vi "总氮质控流程.vi"(6 "队列输入TN":refnum<queue>, 9 "总氮":bool, 10 "总氮量程切换":enum32{"H", "L", "AUTO"}(ring)=enum."AUTO") -> (2 "总氮中断报警":bool, 3 "布尔":bool)   [LabVIEW 2016]
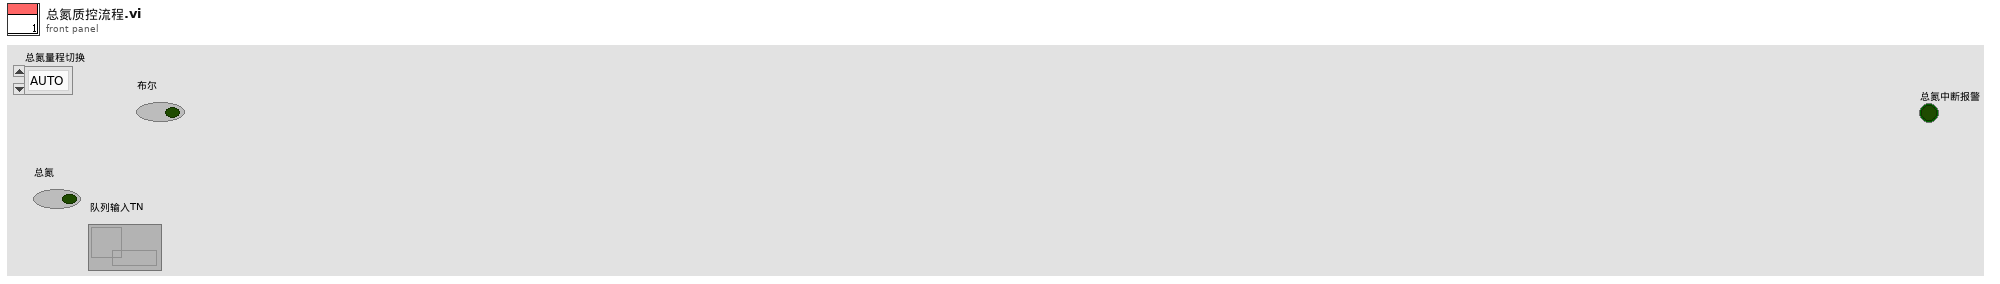
[diagram p1: front panel]
types:
  T1 = enum16{"待机", "启动氨氮水样", "氨氮测量中", "启动氨氮加标", "启动氨氮加标回收", "氨氮加标回收测量中", "启动总氮水样", "总氮测量中", "启动总氮加标", "启动总氮加标回收", "总氮加标回收测量中", "启动总磷水样", "总磷水样测量中", "启动总磷加标", "启动总磷加标回收", "总磷加标回收测量中", "结束"}
  T2 = cluster{"站号":u16, "量程切换":enum32{"H", "L", "AUTO"}, "控制命令":enum16{"启动测量", "标样核查", "零点核查", "跨度核查", "空白测试", "平行样测试", "加标回收", "空白校准", "标样校准", "初始化（清洗）", "停止测试", "仪器重启", "校时", "模式设置", "测量间隔设置"}, "模式设置":enum16{"待机", "连续模式", "周期模式", "定点模式", "受控模式", "手动模式"}, "测量间隔":u16}
  T3 = cluster{"时间标识":timestamp, "设备":string, "日志信息":string}
  T4 = cluster{"系统时间":timestamp, "工作状态":enum16{"空闲", "水样测试", "标样核查", "零点核查", "跨度核查", "空白测试", "平行样测试", "加标回收", "空白校准", "标样校准", "初始化（清洗）"}, "测量模式":enum16{"待机", "连续模式", "周期模式", "定点模式", "受控模式", "手动模式"}, "告警代码":enum16{"无告警", "缺试剂告警", "缺水样告警", "缺蒸馏水告警", "缺标液告警", "仪表漏液告警", "标定异常告警", "超量程告警", "加热异常", "低试剂预警", "超上限告警", "超下限告警", "仪表内部其他异常", "滴定异常告警", "电极异常告警", "量程切换告警", "参数设置告警", "PH电极电位异常", "电导率电极异常", "浊度光度异常", "溶解氧电极异常", "溶解氧光强异常", "温度异常告警", "PH异常告警", "溶解氧异常告警", "电导率异常告警", "浊度异常告警", "叶绿素异常告警", "藻密度异常告警", "蓝绿藻异常告警", "ORP异常告警", "氨氮异常告警", "清洁刷异常告警", "SD卡异常告警", "蓝牙异常告警", "Wifi异常告警", "流程异常告警"}, "故障代码":enum16{"无故障", "电机故障", "温度故障", "通讯故障", "滴定故障"}, "日志代码":u16, "软件版本":u16, "F0":sgl, "F1":sgl, "F2":sgl, "F3":sgl, "T":sgl, "H":sgl, "id":u16, "flowid":u16, "量程":u16, "总磷控温温度1":sgl, "营养盐控温温度2":sgl, "ADC":sgl}
  T5 = enum16{"空闲", "水样测试", "标样核查", "零点核查", "跨度核查", "空白测试", "平行样测试", "加标回收", "空白校准", "标样校准", "初始化（清洗）"}
  T6 = cluster{"因子编码":u32, "单位":u16, "标样参考值":sgl, "水样数据时间":timestamp, "水样实测值":sgl, "水样数据标识":string, "标样数据时间":timestamp, "标样实测值":sgl, "标样数据标识":string, "空白数据时间":timestamp, "空白实测值":sgl, "空白数据标识":string, "零点核查数据时间":timestamp, "零点核查实测值":sgl, "零点核查数据标识":string, "跨度核查数据时间":timestamp, "跨度核查实测值":sgl, "跨度核查数据标识":string, "加标回收数据时间":timestamp, "加标回收实测值":sgl, "加标回收数据标识":string, "平行样数据时间":timestamp, "平行样实测值":sgl, "平行样数据标识":string}
  T7 = cluster{"量程":dbl, "检出限":dbl, "加标前水样浓度":dbl, "加标后水样浓度":dbl, "加标水杯定容体积":dbl, "加标母液浓度":dbl, "加标体积":dbl, "加标回收率":dbl}
  T8 = cluster{"氨氮":u8, "总磷":u8, "总氮":u8, "CODMn":u8, "CODCr":u8}
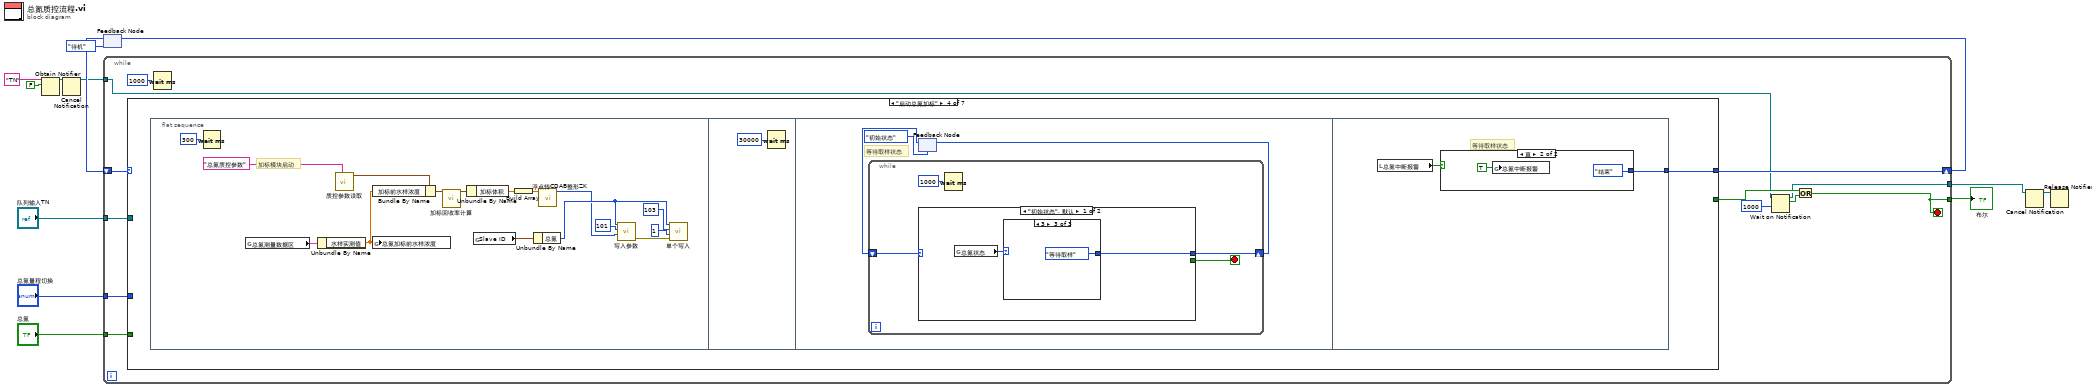
[diagram p0: block diagram]
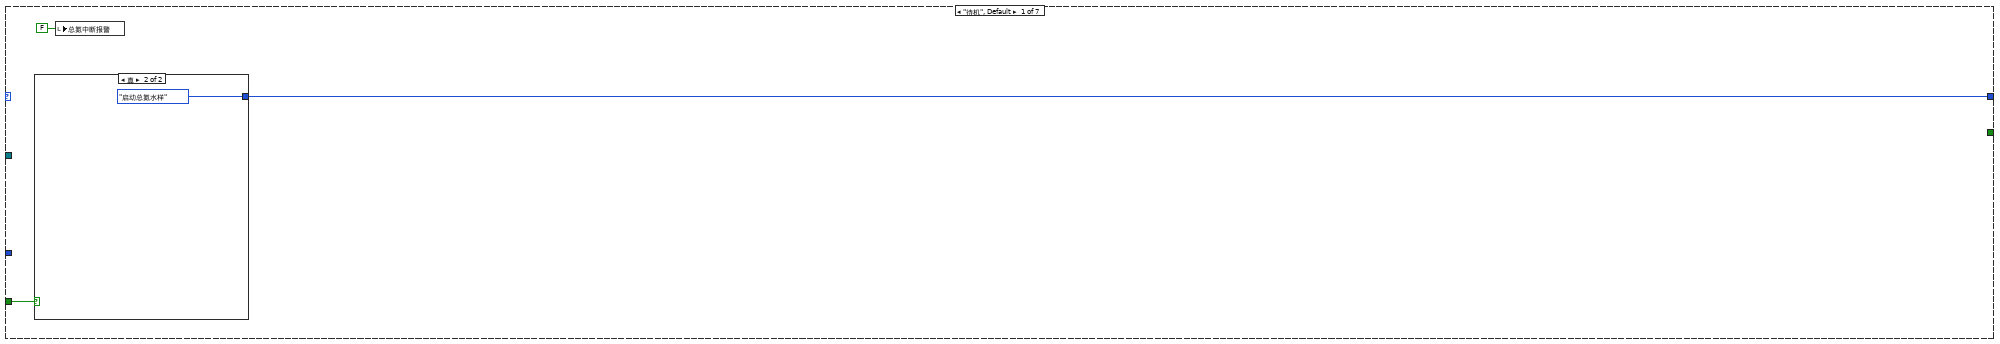
[diagram p2: hidden frame]
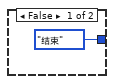
[diagram p3: hidden frame]
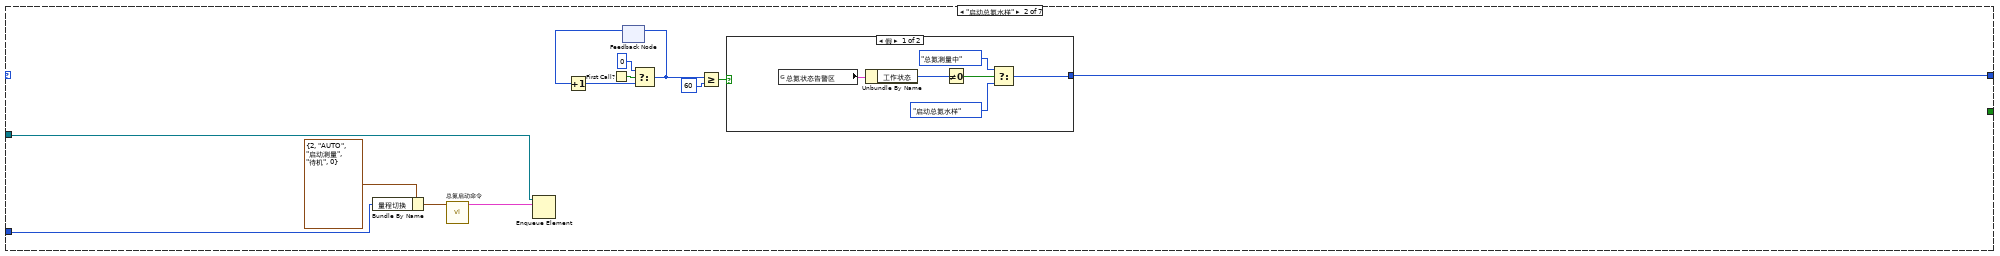
[diagram p4: hidden frame]
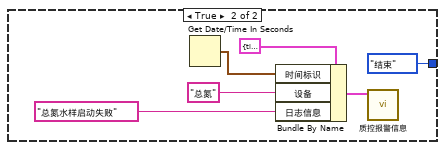
[diagram p5: hidden frame]
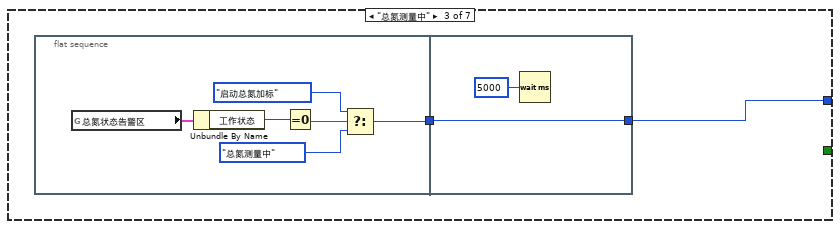
[diagram p6: hidden frame]
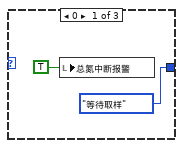
[diagram p7: hidden frame]
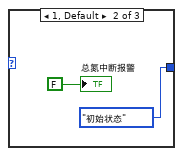
[diagram p8: hidden frame]
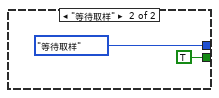
[diagram p9: hidden frame]
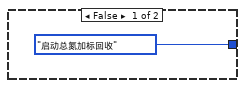
[diagram p10: hidden frame]
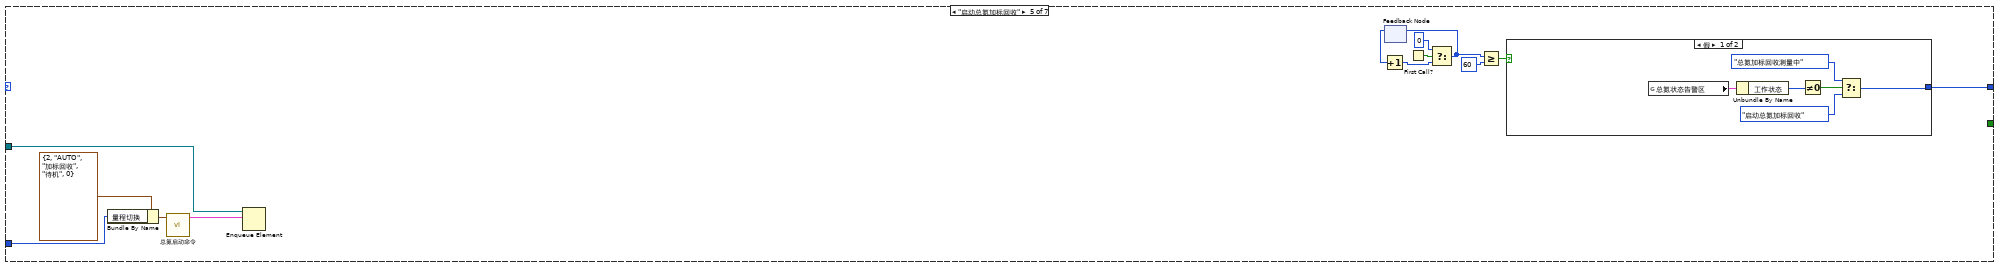
[diagram p11: hidden frame]
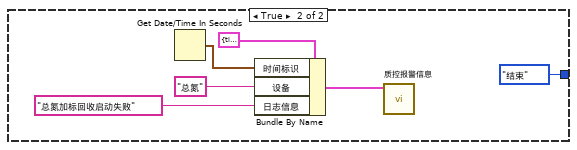
[diagram p12: hidden frame]
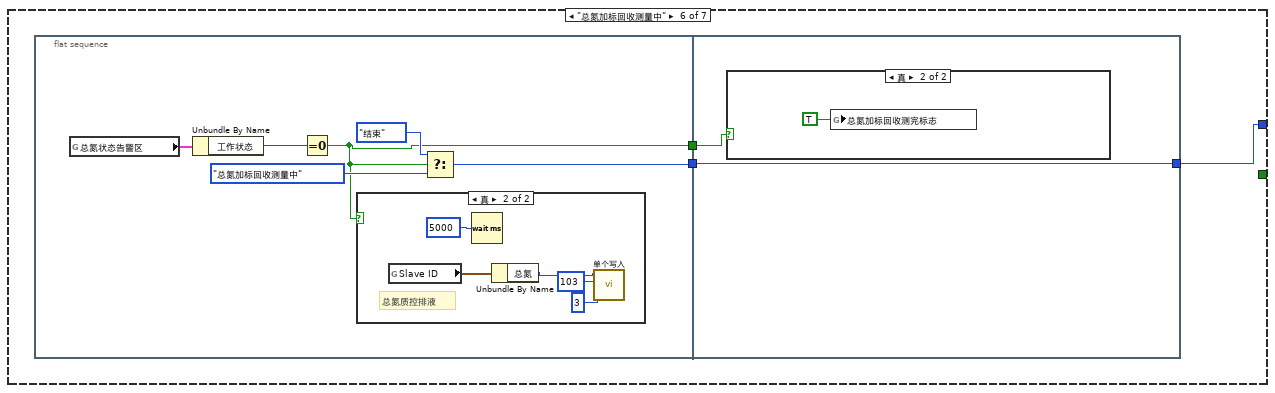
[diagram p13: hidden frame]
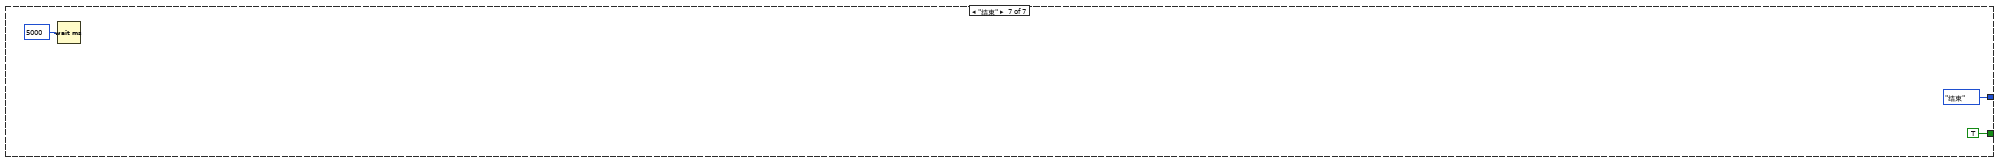
[diagram p16: hidden frame]
diagram:
  n1 = Obtain Notifier(name (unnamed)="TN" ("名称（未命名）"), notification data type=FALSE) -> (notifier out=w4:refnum<notifier>)  [unwired: 2 in, 2 out]
  n2 = Cancel Notification(0:w4) -> (8:w1:refnum<notifier>)  [unwired: 1 in, 2 out]
  n3 = feedback #1(T1."待机") -> (w7:T1)
  n4 = while {
    tunnel: "队列输入TN" -> [w23]
    tunnel: "总氮量程切换" -> [w22]
    tunnel: "总氮" -> [w25]
    tunnel: [w17] -> w12
    shift-right: [w24] -> w10
    shift-left: w7 -> [w21]
    tunnel: w1 -> [w15]
    tunnel: [w16] -> w2
    stop <- w17 stop-if-true
    n5 = case shown="\"启动总氮加标\"" w21 {
      tunnel: [w28 w43 w56 w66 w110 w131 T1."结束"] -> w24
      tunnel: [_ _ _ _ _ _ TRUE] -> w18
      tunnel: w25 -> [w27 _ _ _ _ _ _]
      tunnel: w23 -> [_ w42 _ _ w109 _ _]
      tunnel: w22 -> [_ w41 _ _ w106 _ _]
      frame "待机", Default {
        n6 = case shown="真" w27 {
          tunnel: [T1."结束" T1."启动总氮水样"] -> w28
          frame False {
          }
          frame True {
          }
        }
        n7 = local write "总氮中断报警"(FALSE ("氨氮中断报警")) -> ()
      }
      frame "启动总氮水样" {
        n8 = Bundle By Name(cluster=T2 {"站号"=2, "量程切换"=enum."AUTO", "控制命令"=enum."启动测量", "模式设置"=enum."待机", "测量间隔"=0} ("参数"), "量程切换"=w41) -> (w33:T2)
        n9 = call "总氮启动命令.vi"("参数"=w33) -> ("启动命令"=w31:cluster{"命令":string, "data":variant})  [unwired: 10 in]
        n10 = Enqueue Element(queue=w42, element=w31) -> ()  [unwired: 2 in, 3 out]
        n11 = First Call?() -> (First Call?: T/F=w39:bool)
        n12 = feedback #2() -> (w38:i32)  [unwired: 1 in]
        n13 = Increment(x=w38) -> (x+1=w37:i32)
        n14 = Select(t=0, s=w39, f=w37) -> (s? t:f=w36:i32)
        n15 = feedback-in #2(w36) -> ()
        n16 = Greater Or Equal?(x=w36, y=60) -> (x >= y?=w34:bool)
        n17 = case shown="假" w34 {
          tunnel: [w48 T1."结束"] -> w43
          frame False {
            n18 = global read "与总氮交互全局.vi" "总氮状态告警区"() -> (w45:T4)
            n19 = Unbundle By Name(w45) -> ("工作状态"=w44:T5)
            n20 = Not Equal To 0?(x=w44) -> (x != 0?=w49:bool)
            n21 = Select(t=T1."总氮测量中", s=w49, f=T1."启动总氮水样") -> (s? t:f=w48:T1)
          }
          frame True {
            n22 = Get Date/Time In Seconds() -> (seconds since 1Jan1904=w55:timestamp)
            n23 = Bundle By Name(cluster=T3 {"时间标识"=timestamp(0 s since 1904-01-01), "设备"="", "日志信息"=""} ("data in"), "时间标识"=w55, "设备"="总氮", "日志信息"="总氮水样启动失败") -> (w50:T3)
            n24 = call "质控报警信息.vi"("data in"=w50) -> ()  [unwired: 11 in]
          }
        }
      }
      frame "总氮测量中" {
        n25 = flat-sequence {
          tunnel: [w58] -> w57
          tunnel: w57 -> [w64]
          tunnel: [w64] -> w56
          frame #0 {
            n26 = global read "与总氮交互全局.vi" "总氮状态告警区"() -> (w63:T4)
            n27 = Unbundle By Name(w63) -> ("工作状态"=w62:T5)
            n28 = Equal To 0?(x=w62) -> (x = 0?=w61:bool)
            n29 = Select(t=T1."启动总氮加标", s=w61, f=T1."总氮测量中") -> (s? t:f=w58:T1)
          }
          frame #1 {
            n30 = Wait (ms)(milliseconds to wait=u32 5000 ("等待时间（毫秒）")) -> ()  [unwired: 1 out]
          }
        }
      }
      frame "启动总氮加标" {
        n31 = flat-sequence {
          tunnel: [w101] -> w66
          frame #0 {
            # "加标模块启动"
            n32 = Wait (ms)(milliseconds to wait=u32 300 ("等待时间（毫秒）")) -> ()  [unwired: 1 out]
            n33 = global read "与总氮交互全局.vi" "总氮测量数据区"() -> (w75:T6)
            n34 = Unbundle By Name(w75) -> ("水样实测值"=w77:sgl)
            n35 = call "质控参数读取.vi"("section"="总氮质控参数") -> ("参数"=w80:T7)  [unwired: 9 in, 1 out]
            n36 = Bundle By Name(cluster=w80, "加标前水样浓度"=w77) -> (w81:T7)
            n37 = global write "水样浓度全局.vi" "总氮加标前水样浓度"(w77) -> ()
            n38 = call "加标回收率计算.vi"("参数"=w81) -> ("参数 out"=w79:T7)  [unwired: 9 in, 1 out]
            n39 = Unbundle By Name(w79) -> ("加标体积"=w78:dbl)
            n40 = global read "断电保存全局.vi" "Slave ID"() -> (w73:T8)
            n41 = Build Array(w78) -> (w74:dbl[])
            n42 = Unbundle By Name(w73) -> ("总氮"=w68:u8)
            n43 = call "浮点转CDAB整形ZK.vi"("浮点数"=w74) -> ("CDAB整形输出"=w67:u16[])  [unwired: 10 in]
            n44 = call "写入参数.vi"("values"=w67, "starting address"=u16 101, "Slave ID"=w68) -> ("error out"=w72:errorcluster)  [unwired: 8 in]
            n45 = call "单个写入.vi"("Error in"=w72, "value"=u16 1, "address"=u16 103, "Slave ID"=w68) -> ()  [unwired: 7 in, 1 out]
          }
          frame #1 {
            n46 = Wait (ms)(milliseconds to wait=u32 30000 ("等待时间（毫秒）")) -> ()  [unwired: 1 out]
          }
          frame #2 {
            # "等待取样状态"
            n47 = feedback #3(enum16{"初始状态", "等待取样"}."初始状态") -> (w85:enum16{"初始状态", "等待取样"})
            n48 = while {
              shift-right: [w89] -> w86
              shift-left: w85 -> [w90]
              stop <- w88 stop-if-true
              n49 = case shown="\"初始状态\", 默认" w90 {
                tunnel: [w92 enum16{"初始状态", "等待取样"}."等待取样"] -> w89
                tunnel: [_ TRUE] -> w88
                frame "初始状态", Default {
                  n50 = global read "加标回收状态全局变量.vi" "总氮状态"() -> (w91:u16)
                  n51 = case shown="3" w91 {
                    tunnel: [enum16{"初始状态", "等待取样"}."等待取样" enum16{"初始状态", "等待取样"}."初始状态" enum16{"初始状态", "等待取样"}."等待取样"] -> w92
                    frame 0 {
                      n52 = local write "总氮中断报警"(TRUE ("氨氮中断报警")) -> ()
                    }
                    frame 1, Default {
                      "总氮中断报警" <- FALSE ("总氮中断报警")
                    }
                    frame 3 {
                    }
                  }
                }
                frame "等待取样" {
                }
              }
              n53 = Wait (ms)(milliseconds to wait=u32 1000 ("等待时间（毫秒）")) -> ()  [unwired: 1 out]
            }
            n54 = feedback-in #3(w86) -> ()
          }
          frame #3 {
            # "等待取样状态"
            n55 = local read "总氮中断报警"() -> (w100:bool)
            n56 = case shown="真" w100 {
              tunnel: [T1."启动总氮加标回收" T1."结束"] -> w101
              frame False {
              }
              frame True {
                n57 = global write "质控中断报警全局.vi" "总氮中断报警"(TRUE ("总氮中断报警")) -> ()
              }
            }
          }
        }
      }
      frame "启动总氮加标回收" {
        n58 = Bundle By Name(cluster=T2 {"站号"=2, "量程切换"=enum."AUTO", "控制命令"=enum."加标回收", "模式设置"=enum."待机", "测量间隔"=0} ("参数"), "量程切换"=w106) -> (w108:T2)
        n59 = call "总氮启动命令.vi"("参数"=w108) -> ("启动命令"=w105:cluster{"命令":string, "data":variant})  [unwired: 10 in]
        n60 = Enqueue Element(queue=w109, element=w105) -> ()  [unwired: 2 in, 3 out]
        n61 = feedback #4() -> (w115:i32)  [unwired: 1 in]
        n62 = Increment(x=w115) -> (x+1=w114:i32)
        n63 = First Call?() -> (First Call?: T/F=w116:bool)
        n64 = Select(t=0, s=w116, f=w114) -> (s? t:f=w113:i32)
        n65 = feedback-in #4(w113) -> ()
        n66 = Greater Or Equal?(x=w113, y=60) -> (x >= y?=w111:bool)
        n67 = case shown="假" w111 {
          tunnel: [w121 T1."结束"] -> w110
          frame False {
            n68 = global read "与总氮交互全局.vi" "总氮状态告警区"() -> (w118:T4)
            n69 = Unbundle By Name(w118) -> ("工作状态"=w123:T5)
            n70 = Not Equal To 0?(x=w123) -> (x != 0?=w122:bool)
            n71 = Select(t=T1."总氮加标回收测量中", s=w122, f=T1."启动总氮加标回收") -> (s? t:f=w121:T1)
          }
          frame True {
            n72 = Get Date/Time In Seconds() -> (seconds since 1Jan1904=w129:timestamp)
            n73 = Bundle By Name(cluster=T3 {"时间标识"=timestamp(0 s since 1904-01-01), "设备"="", "日志信息"=""} ("data in"), "时间标识"=w129, "设备"="总氮", "日志信息"="总氮加标回收启动失败") -> (w124:T3)
            n74 = call "质控报警信息.vi"("data in"=w124) -> ()  [unwired: 11 in]
          }
        }
      }
      frame "总氮加标回收测量中" {
        n75 = flat-sequence {
          tunnel: [w137] -> w132
          tunnel: [w133] -> w130
          tunnel: [w145] -> w131
          tunnel: w132 -> [w145]
          tunnel: w130 -> [w144]
          frame #0 {
            n76 = global read "与总氮交互全局.vi" "总氮状态告警区"() -> (w134:T4)
            n77 = Unbundle By Name(w134) -> ("工作状态"=w138:T5)
            n78 = Equal To 0?(x=w138) -> (x = 0?=w133:bool)
            n79 = case shown="真" w133 {
              frame False {
              }
              frame True {
                # "总氮质控排液"
                n80 = global read "断电保存全局.vi" "Slave ID"() -> (w142:T8)
                n81 = Wait (ms)(milliseconds to wait=u32 5000 ("等待时间（毫秒）")) -> ()  [unwired: 1 out]
                n82 = Unbundle By Name(w142) -> ("总氮"=w139:u8)
                n83 = call "单个写入.vi"("value"=u16 3, "address"=u16 103, "Slave ID"=w139) -> ()  [unwired: 8 in, 1 out]
              }
            }
            n84 = Select(t=T1."结束", s=w133, f=T1."总氮加标回收测量中") -> (s? t:f=w137:T1)
          }
          frame #1 {
            n85 = case shown="真" w144 {
              frame False {
              }
              frame True {
                n86 = global write "质控测完标志全局 1.vi" "总氮加标回收测完标志"(TRUE) -> ()
              }
            }
          }
        }
      }
      frame "结束" {
        n87 = Wait (ms)(milliseconds to wait=u32 5000 ("等待时间（毫秒）")) -> ()  [unwired: 1 out]
      }
    }
    n88 = Wait (ms)(milliseconds to wait=u32 1000 ("等待时间（毫秒）")) -> ()  [unwired: 1 out]
    n89 = Wait on Notification(notifier=w15, timeout in ms (-1)=1000 ("超时毫秒(-1)")) -> (notifier out=w16:refnum<notifier>, notification=w19:bool)  [unwired: 2 in, 2 out]
    n90 = Or(x=w18, y=w19) -> (x .or. y?=w17:bool)
  }
  "布尔" <- w12
  n91 = feedback-in #1(w10) -> ()
  n92 = Cancel Notification(0:w2) -> (8:w3:refnum<notifier>)  [unwired: 1 in, 2 out]
  n93 = Release Notifier(notifier=w3) -> ()  [unwired: 2 in, 3 out]
